vi "ParseSWI.vi"(8 "error in (no error)":errorcluster, 9 "Master Device in":refnum<class "Master Device.lvclass">, 10 "Current Variables":T1[](array[typedef]), 11 "Aerotech_Soloist in":refnum<class "Aerotech_Soloist.lvclass">) -> (0 "error out":errorcluster, 2 "Master Device out":refnum<class "Master Device.lvclass">, 3 "Aerotech_Soloist out":refnum<class "Aerotech_Soloist.lvclass">)   [LabVIEW 2013, in "Aerotech_Soloist.lvclass"]
doc: "All specific devices will override ParseSWI method (i.e. you can delete the parent call)\n (1) Get devices data from private data\n (2) Get Slave Info (Ramp List) from Master Device\n (3) Parse data into \"prepared HWI\" which is in reverse order to match Ramp List."
uses:
  Aerotech_Soloist.lvclass
  TypeDefs/Active procedure variables.ctl
  Master Device/Master Device.lvclass
  ColumnVIs/MenuCol/MenuCol.lvclass
  ParsedSWILine.ctl
  Aerotech_Soloist.lvclass/Aerotech_Soloist.ctl
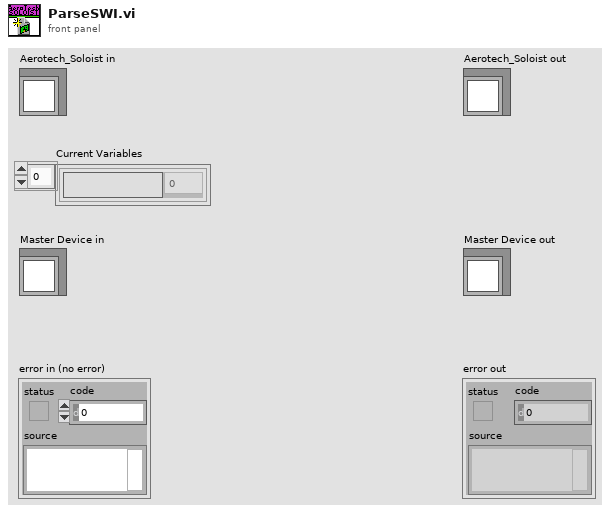
[diagram p1: front panel]
types:
  T1 = typedef "Active procedure variables.ctl" = cluster{"Procedure variable":string, "Value":dbl}
  T2 = typedef "Aerotech_Soloist.lvclass/ParsedSWILine.ctl" = cluster{"ParameterScript":string, "CommandScript":string}
  T3 = typedef "SlaveInfo.ctl" = cluster{"Triggering":bool[][], "Ramp Info":T4[], "Line Inversion":bool[], "Slaved Digital Channels":cluster{"Master Channel Number":i32, "Output States":bool[]}[]}
  T4 = typedef "RampInfo.ctl" = cluster{"Table Ramp Index":i32, "Ramp Time":dbl, "Number of Steps":i32, "Instruction Array Index":i32}
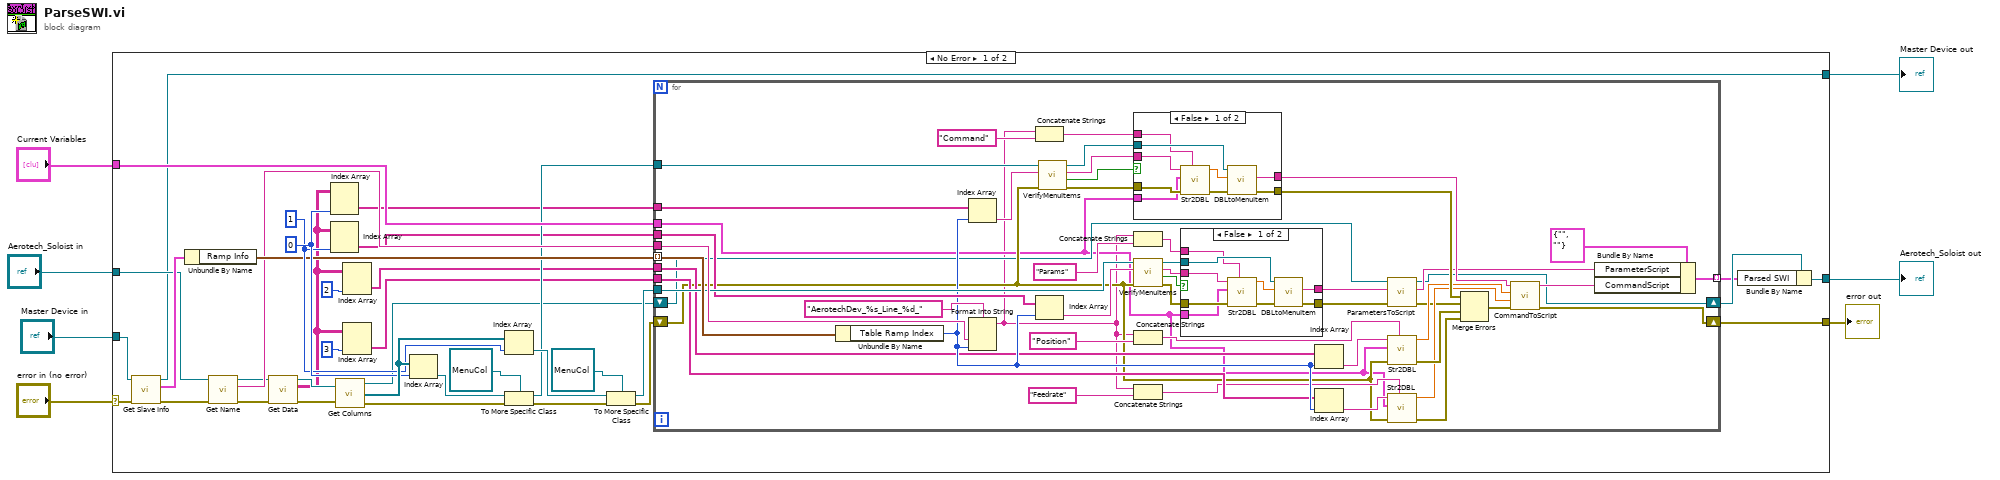
[diagram p0: block diagram]
diagram:
  n1 = case shown="No Error" "error in (no error)" {
    selector: "error in (no error)" -> [w43 w117]
    tunnel: "Master Device in" -> [w44 w118]
    tunnel: "Aerotech_Soloist in" -> [w25 w119]
    tunnel: "Current Variables" -> [w30 _]
    tunnel: [w13 w118] -> w3
    tunnel: [w10 w119] -> w2
    tunnel: [w11 w117] -> w1
    frame No Error {
      w32 = 1 ("index")
      w33 = 0 ("index")
      n2 = call-dynamic "Get Slave Info.vi"("error in (no error)"=w43, "Master Device in"=w44) -> ("error out"=w26:errorcluster, "Slave Info"=w40:T3, "Master Device out"=w13:refnum<class "Master Device.lvclass">)  [unwired: 7 in]
      n3 = Unbundle By Name(w40) -> ("Ramp Info"=w29:T4[])
      n4 = call-dynamic "Get Name.vi"("error in (no error)"=w26, "Device in"=w25) -> ("error out"=w23:errorcluster, "Name"=w28:string, "Device out"=w24:refnum<class "Aerotech_Soloist.lvclass">)  [unwired: 7 in]
      n5 = call-dynamic "Get Data.vi"("error in (no error)"=w23, "Device in"=w24) -> ("error out"=w41:errorcluster, "Table Indicator"=w18:string[][], "Device out"=w42:refnum<class "Aerotech_Soloist.lvclass">)  [unwired: 6 in]
      n6 = Index Array(array=w18, index (col)=w33) -> (element=w20:string[])  [unwired: 1 in]
      n7 = Index Array(array=w18, index (col)=w32) -> (element=w19:string[])  [unwired: 1 in]
      n8 = call-dynamic "Get Columns.vi"("Device in"=w42, "error in (no error)"=w41) -> ("Device out"=w12:refnum<class "Aerotech_Soloist.lvclass">, "Columns"=w34:refnum<class "Column.lvclass">[], "error out"=w27:errorcluster)
      n9 = Index Array(array=w18, index (col)=2 ("disabled index (col)")) -> (element=w15:string[])  [unwired: 1 in]
      n10 = Index Array(array=w18, index (col)=3 ("disabled index (col)")) -> (element=w14:string[])  [unwired: 1 in]
      n11 = Index Array(array=w34, index=w33) -> (element=w38:refnum<class "Column.lvclass">)
      n12 = Index Array(array=w34, index=w32) -> (element=w37:refnum<class "Column.lvclass">)
      n13 = To More Specific Class(target class=refnum<class "MenuCol.lvclass"> refnum ("MenuCol.lvclass"), reference=w38, error in=w27) -> (specific class reference=w22:refnum<class "MenuCol.lvclass">, error out=w35:errorcluster)
      n14 = To More Specific Class(target class=refnum<class "MenuCol.lvclass"> refnum ("MenuCol.lvclass"), reference=w37, error in=w35) -> (specific class reference=w21:refnum<class "MenuCol.lvclass">, error out=w31:errorcluster)
      n15 = for {
        tunnel: w15 -> [w80]
        shift-right: [w65] -> w11
        shift-left: w31 -> [w64]
        tunnel: w30 -> [w52]
        tunnel: w29 -> [w94] mode=indexing
        tunnel: w28 -> [w92]
        tunnel: w22 -> [w91]
        tunnel: w21 -> [w90]
        tunnel: w20 -> [w89]
        tunnel: w19 -> [w82]
        tunnel: w14 -> [w79]
        tunnel: [w62] -> w8 mode=indexing
        shift-right: [w58] -> w9
        shift-left: w12 -> [w57]
        n16 = Unbundle By Name(w94) -> ("Table Ramp Index"=w81:i32)
        n17 = Index Array(array=w89, index=w81) -> (element=w88:string)
        n18 = Format Into String(format string="AerotechDev_%s_Line_%d_", w92, w81) -> (resulting string=w47:string)  [unwired: 2 in, 1 out]
        n19 = Concatenate Strings(w47, "Command" ("string")) -> (w54:string)
        n20 = Index Array(array=w82, index=w81) -> (element=w83:string)
        n21 = call-dynamic "VerifyMenuItems.vi"("error in (no error)"=w64, "Menu Item In"=w88, "MenuCol in"=w91) -> ("error out"=w85:errorcluster, "Valid Menu Item"=w87:bool, "Menu Item Out"=w84:string, "MenuCol out"=w86:refnum<class "MenuCol.lvclass">)  [unwired: 5 in]
        n22 = case shown="False" w87 {
          tunnel: w86 -> [w114 _]
          tunnel: w85 -> [w110 w115]
          tunnel: w84 -> [w108 w116]
          tunnel: [w112 w116] -> w69
          tunnel: [w113 w115] -> w70
          tunnel: w54 -> [w107 _]
          tunnel: w52 -> [w106 _]
          frame False {
            n23 = call "Str2DBL.vi"("Error Locator"=w107, "error in (no error)"=w110, "Current Variable settings"=w106, "formula"=w108) -> ("error out"=w111:errorcluster, "y value"=w109:dbl)  [unwired: 4 in]
            n24 = call-dynamic "DBLtoMenuItem.vi"("error in (no error)"=w111, "Double In"=w109, "MenuCol in"=w114) -> ("error out"=w113:errorcluster, "Menu Item"=w112:string)  [unwired: 6 in, 1 out]
          }
          frame True {
          }
        }
        n25 = Concatenate Strings(w47, "Params" ("string")) -> (w48:string)
        n26 = call-dynamic "VerifyMenuItems.vi"("error in (no error)"=w64, "Menu Item In"=w83, "MenuCol in"=w90) -> ("error out"=w53:errorcluster, "Valid Menu Item"=w50:bool, "Menu Item Out"=w51:string, "MenuCol out"=w49:refnum<class "MenuCol.lvclass">)  [unwired: 5 in]
        n27 = Concatenate Strings(w47, "Position" ("string")) -> (w76:string)
        n28 = Concatenate Strings(w47, "Feedrate" ("string")) -> (w75:string)
        n29 = case shown="False" w50 {
          tunnel: w49 -> [w103 _]
          tunnel: w53 -> [w99 w104]
          tunnel: w51 -> [w97 w105]
          tunnel: [w101 w105] -> w46
          tunnel: [w102 w104] -> w45
          tunnel: w48 -> [w96 _]
          tunnel: w52 -> [w95 _]
          frame False {
            n30 = call "Str2DBL.vi"("Error Locator"=w96, "error in (no error)"=w99, "Current Variable settings"=w95, "formula"=w97) -> ("error out"=w100:errorcluster, "y value"=w98:dbl)  [unwired: 4 in]
            n31 = call-dynamic "DBLtoMenuItem.vi"("error in (no error)"=w100, "Double In"=w98, "MenuCol in"=w103) -> ("error out"=w102:errorcluster, "Menu Item"=w101:string)  [unwired: 6 in, 1 out]
          }
          frame True {
          }
        }
        n32 = Index Array(array=w80, index=w81) -> (element=w77:string)
        n33 = Index Array(array=w79, index=w81) -> (element=w78:string)
        n34 = call-dynamic "ParametersToScript.vi"("error in (no error)"=w45, "Params In"=w46, "Aerotech_Soloist in"=w57) -> ("error out"=w60:errorcluster, "AeroBasic Template Out"=w59:string, "Aerotech_Soloist out"=w58:refnum<class "Aerotech_Soloist.lvclass">)  [unwired: 6 in]
        n35 = call "Str2DBL.vi"("Error Locator"=w76, "error in (no error)"=w64, "Current Variable settings"=w52, "formula"=w77) -> ("error out"=w71:errorcluster, "y value"=w68:dbl)  [unwired: 4 in]
        n36 = call "Str2DBL.vi"("Error Locator"=w75, "error in (no error)"=w64, "Current Variable settings"=w52, "formula"=w78) -> ("error out"=w72:errorcluster, "y value"=w67:dbl)  [unwired: 4 in]
        n37 = Merge Errors(w70, w60, w71, w72) -> (w66:errorcluster)
        n38 = call "CommandToScript.vi"("error in (no error)"=w66, "Feedrate In"=w67, "Position In"=w68, "Command In"=w69) -> ("error out"=w65:errorcluster, "AeroBasic Template Out"=w61:string)  [unwired: 6 in]
        n39 = Bundle By Name(cluster=T2 {"ParameterScript"="", "CommandScript"=""} ("Cluster"), "ParameterScript"=w59, "CommandScript"=w61) -> (w62:T2)
      }
      n40 = Bundle By Name(cluster=w9, "Parsed SWI"=w8) -> (w10:refnum<class "Aerotech_Soloist.lvclass">)
    }
    frame Error {
    }
  }
  "error out" <- w1
  "Aerotech_Soloist out" <- w2
  "Master Device out" <- w3
